vi "NicmosSetFilter.vi"(2 "FILTERCOMMAND":T1, 9 "error in (no error)":errorcluster caption="error out (no error)") -> (6 "error out":errorcluster)   [LabVIEW 2009]
uses:
  Controls/NICMOS.FILTERCOMMAND.ctl
  Controls/NICMOS.FILTER.ctl
  Controls/NICMOS.COMMAND.ctl
  Controls/NICMOS.COMMANDBASIC.ctl
  Controls/NICMOS.READOUT.ctl
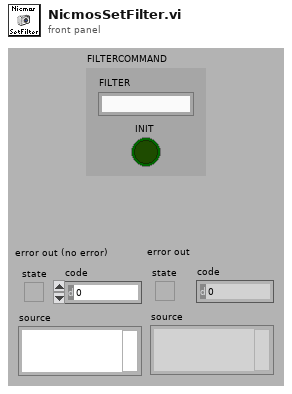
[diagram p1: front panel]
types:
  T1 = typedef "NICMOS.FILTERCOMMAND.ctl" = cluster{"FILTER":T2, "INIT":bool}
  T2 = typedef "NICMOS.FILTER.ctl" = string
  T3 = typedef "NICMOS.COMMAND.ctl" = cluster{"Command":T4, "READOUT":T5, "FILTERCOMMAND":T1, "ACQUISITION":i32, "Done":refnum<k4>}
  T4 = typedef "NICMOS.COMMANDBASIC.ctl" = enum16{"WRITE BANKS", "SET FILTER", "HOME FILTER", "QUERY TEMP", "CONFIGURE", "START", "ACQUISITION", "STOP", "QUIT"}
  T5 = typedef "NICMOS.READOUT.ctl" = cluster{"Readout":i32, "Deglitch":i32, "Framerate":dbl[unit], "Bank":i32}
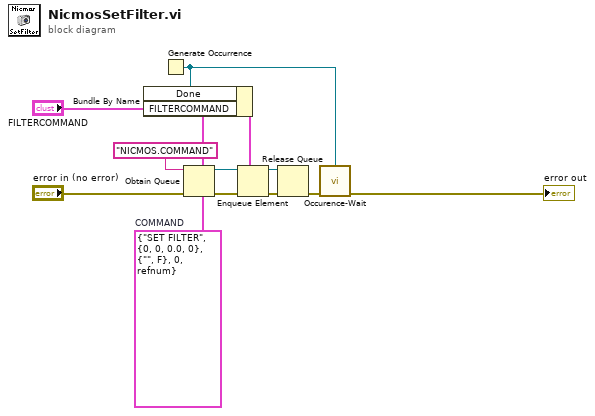
[diagram p0: block diagram]
diagram:
  w8 = T3 {"Command"=enum."SET FILTER", "READOUT"={"Readout"=0, "Deglitch"=0, "Framerate"=0.0, "Bank"=0}, "FILTERCOMMAND"={"FILTER"="", "INIT"=FALSE}, "ACQUISITION"=0, "Done"=refnum}  # COMMAND
  n1 = Generate Occurrence() -> (w6:refnum<k4>)
  n2 = Bundle By Name(cluster=w8, "Done"=w6, "FILTERCOMMAND"="FILTERCOMMAND") -> (w9:T3)
  n3 = Obtain Queue(name (unnamed)="NICMOS.COMMAND" ("nom (aucun)"), element data type=w8, error in (no error)="error in (no error)") -> (queue out=w5:refnum<queue>, error out=w3:errorcluster)  [unwired: 2 in, 1 out]
  n4 = Enqueue Element(queue=w5, element=w9, error in (no error)=w3) -> (queue out=w4:refnum<queue>, error out=w11:errorcluster)  [unwired: 1 in, 1 out]
  n5 = Release Queue(queue=w4, error in (no error)=w11) -> (error out=w7:errorcluster)  [unwired: 1 in, 2 out]
  n6 = call "Occurence-Wait.vi"("occurrence"=w6, "error out"=w7) -> ("error in (no error)"=→"error out":errorcluster)  [unwired: 7 in]
